vi "Handle Error.vi"(8 "error in (no error)":errorcluster, 11 "Function UI in":refnum<class "Controller UI.lvclass">) -> (0 "error out":errorcluster, 2 "stop actor?":bool=TRUE, 3 "Function UI out":refnum<class "Controller UI.lvclass">)   [LabVIEW 2016, in "Controller UI.lvlib" / "Controller UI.lvclass"]
doc: "(<B>Filename</B>: Actor Framework.lvlib:Actor.lvclass:Handle Error.vi)\n\nDefines how the actor handles an error that occurred while processing a message.\n\nBy default, this method does nothing except stop the actor. This method also treats error code 43 (coming from <B>error in</B>) as a sign that the actor shut down normally. In this situation, the Handle Error method does not return the error on <B>error out</B>, meaning the actor's caller will not receive it. All other error codes will be returned on <B>error out</B>.\n\nA descendant class may override this method to change this behavior."
uses:
  <userlib>/Common Components/Controller UI/Controller UI.lvclass
  C:/Program Files (x86)/National Instruments/LabVIEW 2016/vi.lib/ActorFramework/Actor/Actor.lvclass
  <vilib>/ActorFramework/Actor/Actor.lvclass/Actor.ctl
  <vilib>/ActorFramework/Message Enqueuer/Message Enqueuer.lvclass/Message Enqueuer.ctl
  <vilib>/ActorFramework/Message Enqueuer/Init from Existing Queue.vi
  <vilib>/ActorFramework/Message Enqueuer/Message Enqueuer.lvclass
  <userlib>/Common Components/User Interface/UI.lvclass
  <userlib>/Common Components/User Interface/Messages/Update Status Display/Update Status Display.lvclass
  <vilib>/ActorFramework/Actor/Actor.lvclass
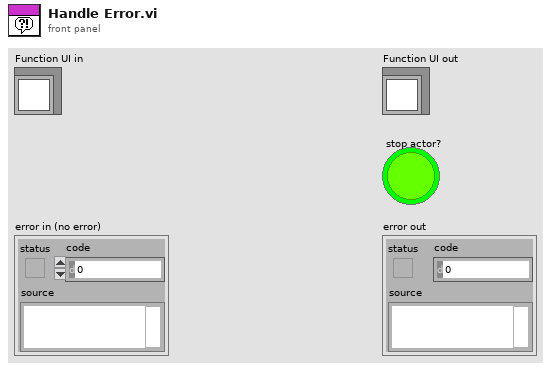
[diagram p1: front panel]
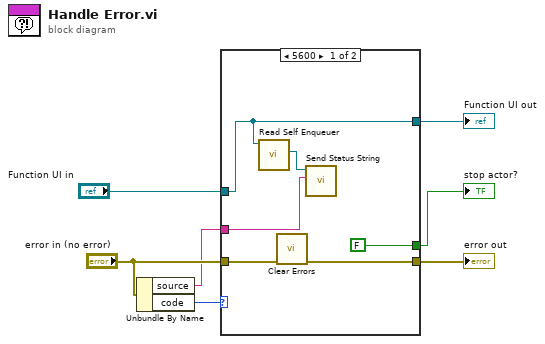
[diagram p0: block diagram]
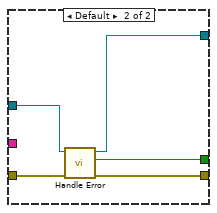
[diagram p2: hidden frame]
diagram:
  n1 = Unbundle By Name("error in (no error)") -> ("source"=w2:string, "code"=w3:i32)
  n2 = case shown="5600" w3 {
    tunnel: [w11 w18] -> w7
    tunnel: [FALSE ("stop actor?") w17] -> w1
    tunnel: [w10 w16] -> w6
    tunnel: "error in (no error)" -> [w12 w15]
    tunnel: "Function UI in" -> [w10 w14]
    tunnel: w2 -> [w8 _]
    frame 5600 {
      n3 = call <vilib>:"Read Self Enqueuer.vi"("Actor"=w10) -> ("Self Enqueuer"=w9:refnum<class "Message Enqueuer.lvclass">)  [unwired: 10 in]
      n4 = call <vilib>:"Clear Errors.vi"("error in (no error)"=w12) -> ("error out"=w11:errorcluster)  [unwired: 5 in, 1 out]
      n5 = call <userlib>:"Send Status String.vi"("String"=w8, "Message Enqueuer in"=w9) -> ()  [unwired: 8 in, 2 out]
    }
    frame Default {
      n6 = call-parent "Handle Error.vi"("error in (no error)"=w15, "UI in"=w14) -> ("error out"=w18:errorcluster, "stop actor?"=w17:bool, "UI out"=w16:refnum<class "Controller UI.lvclass">)  [unwired: 7 in]
    }
  }
  "Function UI out" <- w6
  "error out" <- w7
  "stop actor?" <- w1
